vi "Read debugLevel.vi"(8 "error in (no error)":errorcluster, 11 "TCSDebug in":refnum<class "TCSDebug.lvclass">) -> (0 "error out":errorcluster, 2 "debugLevel":T1, 3 "TCSDebug out":refnum<class "TCSDebug.lvclass">)   [LabVIEW 2022 SP3, in "TCSDataDefinitions.lvlib" / "TCSCommand.lvlib" / "TCSDebug.lvclass"]
uses:
  TCSDebug.lvclass
  Enumerations/TCSDebuLevelTypes.ctl
  TCSDebug.lvclass/TCSDebug.ctl
  TCSCommand.lvlib
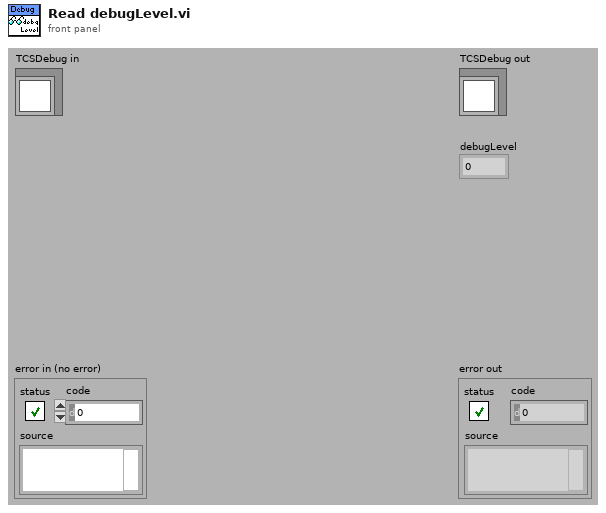
[diagram p1: front panel]
types:
  T1 = typedef "TCSDataDefinitions.lvlib/TCSCommand.lvlib/TCSDebuLevelTypes.ctl" = enum16{"0", "1", "2", "3", "4", "5", "6", "7", "8", "9", "10"}
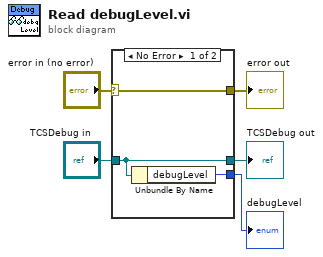
[diagram p0: block diagram]
diagram:
  n1 = case shown="No Error" "error in (no error)" {
    selector: "error in (no error)" -> [w8 w9]
    tunnel: [w8 w9] -> w4
    tunnel: [w7 w10] -> w2
    tunnel: "TCSDebug in" -> [w7 w10]
    tunnel: [w6 _] -> w1
    frame No Error {
      n2 = Unbundle By Name(w7) -> ("debugLevel"=w6:T1)
    }
    frame Error {
    }
  }
  "error out" <- w4
  "TCSDebug out" <- w2
  "debugLevel" <- w1
